vi "niLvFpgaNotchCU(16-bit).vi"(0 "filter state in":T1, 1 "reset":bool, 5 "input data":i16, 7 "y(n-1) from accum":i32, 9 "adder in":i32, 11 "iteration":u8, 12 "in shift":i8=-1) -> (4 "filter state out":T1, 6 "state to multiply":i32, 8 "accumulator out":i32, 10 "adder out":i32, 15 "terminate":bool)   [LabVIEW 2017]
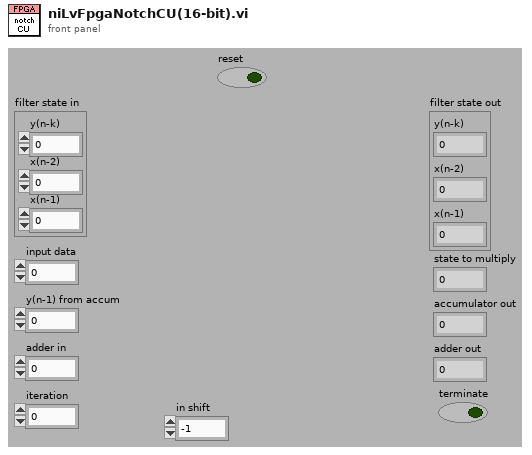
[diagram p1: front panel]
types:
  T1 = cluster{"y(n-k)":i32, "x(n-2)":i16, "x(n-1)":i16}
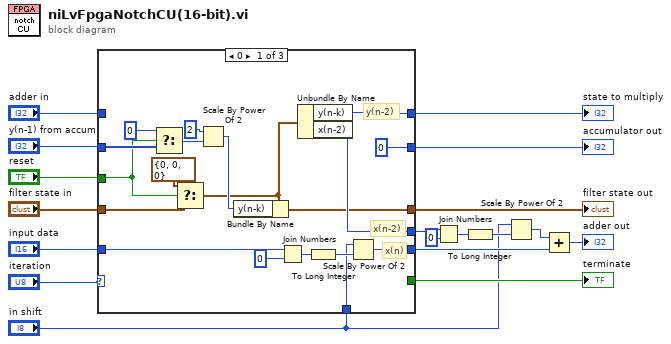
[diagram p0: block diagram]
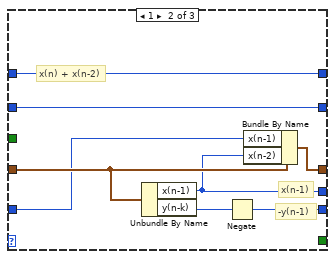
[diagram p2: hidden frame]
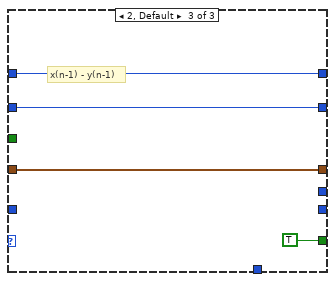
[diagram p3: hidden frame]
diagram:
  n1 = case shown="0" "iteration" {
    tunnel: [w20 w40 w49] -> w15
    tunnel: "filter state in" -> [w22 w41 w49]
    tunnel: "input data" -> [w30 w38 _]
    tunnel: [w34 w43 _] -> w4
    tunnel: "adder in" -> [_ w44 w47]
    tunnel: [w31 w44 w47] -> w14
    tunnel: [w25 w39 _] -> w11
    tunnel: "y(n-1) from accum" -> [w27 w45 w48]
    tunnel: [0 ("Numeric") w45 w48] -> w6
    tunnel: [_ _ TRUE] -> w7
    tunnel: "reset" -> [w24 _ _]
    tunnel: "in shift" -> [w23 _ _]
    frame 0 {
      # "x(n)"
      # "x(n-2)"
      # "y(n-2)"
      n2 = Select(t=0, s=w24, f=w27) -> (s? t:f=w28:i32)
      n3 = Select(t=T1 {"y(n-k)"=0, "x(n-2)"=0, "x(n-1)"=0} ("filter state in"), s=w24, f=w22) -> (s? t:f=w19:T1)
      n4 = Scale By Power Of 2(n=2, x=w28) -> (x*2^n=w26:i32)
      n5 = Bundle By Name(cluster=w19, "y(n-k)"=w26) -> (w20:T1)
      n6 = Join Numbers(hi=w30, lo=i16 0) -> ((hi.lo)=w37:u32)
      n7 = Unbundle By Name(w19) -> ("y(n-k)"=w31:i32, "x(n-2)"=w25:i16)
      n8 = To Long Integer(number=w37) -> (32bit integer=w35:i32)
      n9 = Scale By Power Of 2(n=w23, x=w35) -> (x*2^n=w34:i32)
    }
    frame 1 {
      # "x(n) + x(n-2)"
      # "-y(n-1)"
      # "x(n-1)"
      n10 = Unbundle By Name(w41) -> ("x(n-1)"=w39:i16, "y(n-k)"=w42:i32)
      n11 = Negate(x=w42) -> (-x=w43:i32)
      n12 = Bundle By Name(cluster=w41, "x(n-1)"=w38, "x(n-2)"=w39) -> (w40:T1)
    }
    frame 2, Default {
      # "x(n-1) - y(n-1)"
    }
  }
  "filter state out" <- w15
  "state to multiply" <- w14
  "terminate" <- w7
  "accumulator out" <- w6
  n13 = Join Numbers(hi=w11, lo=i16 0) -> ((hi.lo)=w10:u32)
  n14 = To Long Integer(number=w10) -> (32bit integer=w9:i32)
  n15 = Scale By Power Of 2(n="in shift", x=w9) -> (x*2^n=w12:i32)
  n16 = Add(x=w12, y=w4) -> (x+y=→"adder out":i32)
